vi "To Cleanup Initialize and Close Session Behavior.vi"(11 "initialize and close session behavior":T1) -> (3 "cleanup initialize and close session behavior":T1)   [LabVIEW 2020, in "NI Session Management Instrument.lvlib" / "ISession Factory.lvclass"]
uses:
  ISession Factory.lvclass
  Initialize and Close Session Behavior.ctl
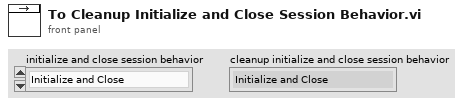
[diagram p1: front panel]
types:
  T1 = typedef "NI Session Management Instrument.lvlib/ISession Factory.lvclass/Initialize and Close Session Behavior.ctl" = enum16{"Initialize and Close", "Attach and Detach", "Initialize and Detach", "Attach and Close"}
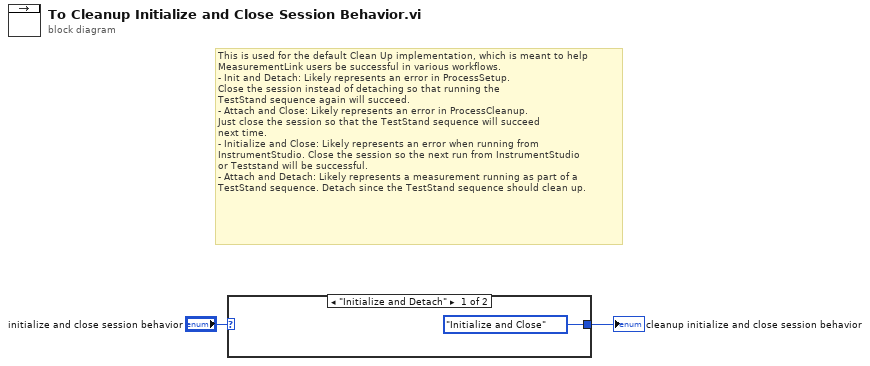
[diagram p0: block diagram]
diagram:
  # "This is used for the default Clean Up implementation, which is meant to help\nMeasurementLink users be successful in various workflows.\n- Init and Detach: Likely represents an error in ProcessSetup.\nClose the session instead of detaching so that running the \nTestStand sequence again will succeed.\n- Attach and Close: Likely represents an error in ProcessCleanup.\nJust close the session so that the TestStand sequence will succeed\nnext time.\n- Initialize and Close: Likely represents an error when running from\nInstrumentStudio. Close the session so the next run from InstrumentStudio\nor Teststand will be successful.\n- Attach and Detach: Likely represents a measurement running as part of a\nTestStand sequence. Detach since the TestStand sequence should clean up."
  n1 = case shown="\"Initialize and Detach\"" "initialize and close session behavior" {
    selector: "initialize and close session behavior" -> [_ w4]
    tunnel: [Initialize_and_Close_Session_Behavior."Initialize and Close" ("cleanup initialize and close session behavior") w4] -> w1
    frame "Initialize and Detach" {
    }
    frame "Initialize and Close", "Attach and Detach", "Attach and Close" {
    }
  }
  "cleanup initialize and close session behavior" <- w1
